vi "Write Data.vi"(10 "Data":i32, 11 "Alpha Task Msg in":refnum<class "Alpha Task Msg.lvclass">) -> (3 "Alpha Task Msg out":refnum<class "Alpha Task Msg.lvclass">)   [LabVIEW 2017, in "Alpha Actor.lvlib" / "Alpha Task Msg.lvclass"]
uses:
  Alpha Task Msg.lvclass
  Alpha Task Msg.lvclass/Alpha Task Msg.ctl
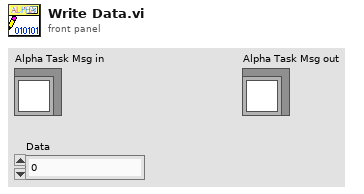
[diagram p1: front panel]
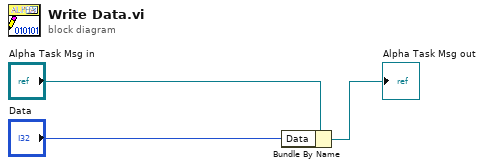
[diagram p0: block diagram]
diagram:
  n1 = Bundle By Name(cluster="Alpha Task Msg in", "Data"="Data") -> (→"Alpha Task Msg out":refnum<class "Alpha Task Msg.lvclass">)
